vi "apend_xwav.vi"(1 "xwave":T1={"attributes"=variant, "X"={"start"=0.0, "delta"=0.0, "units"="index", "dim"="au"}, "Y"={"data"=[], "units"="au"}}, 2 "xwave to append":T1={"attributes"=variant, "X"={"start"=0.0, "delta"=0.0, "units"="index", "dim"="au"}, "Y"={"data"=[], "units"="au"}}) -> (4 "appended?":bool, 6 "xwave out":T1={"attributes"=variant, "X"={"start"=0.0, "delta"=0.0, "units"="index", "dim"="au"}, "Y"={"data"=[], "units"="au"}})   [LabVIEW 2015]
uses:
  xwav.ctl
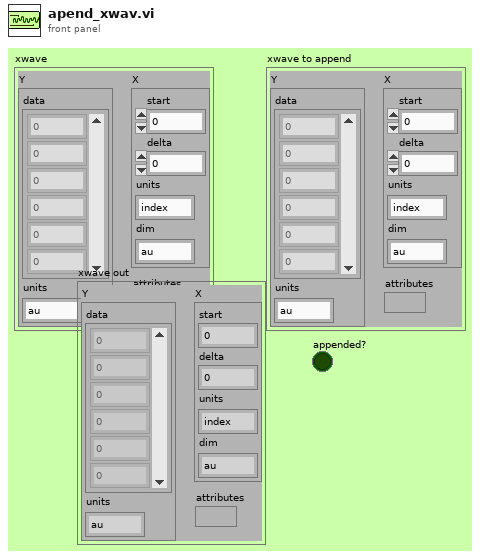
[diagram p1: front panel]
types:
  T1 = typedef "xwav.ctl" = cluster{"attributes":variant, "X":cluster{"start":dbl, "delta":dbl, "units":string, "dim":string}, "Y":cluster{"data":dbl[], "units":string}}
  T2 = cluster{"attributes":bool, "X":cluster{"start":bool, "delta":bool, "units":bool, "dim":bool}, "Y":cluster{"data":bool[], "units":bool}}
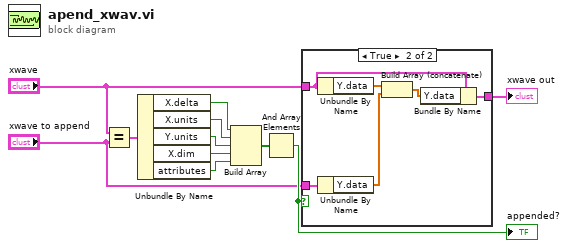
[diagram p0: block diagram]
diagram:
  n1 = Equal?(x="xwave", y="xwave to append") -> (x = y?=w11:T2)
  n2 = Unbundle By Name(w11) -> ("X.delta"=w10:bool, "X.units"=w9:bool, "Y.units"=w8:bool, "X.dim"=w7:bool, "attributes"=w1:bool)
  n3 = Build Array(w10, w9, w8, w7, w1) -> (w6:bool[])
  n4 = And Array Elements(Boolean array=w6) -> (logical AND=w5:bool)
  "appended?" <- w5
  n5 = case shown="True" w5 {
    tunnel: "xwave" -> [w12 w15]
    tunnel: "xwave to append" -> [_ w18]
    tunnel: [w12 w13] -> w2
    frame False {
    }
    frame True {
      n6 = Unbundle By Name(w15) -> ("Y.data"=w17:dbl[])
      n7 = Unbundle By Name(w18) -> ("Y.data"=w16:dbl[])
      n8 = Build Array (concatenate)(w17, w16) -> (w14:dbl[])
      n9 = Bundle By Name(cluster=w15, "Y.data"=w14) -> (w13:T1)
    }
  }
  "xwave out" <- w2
